vi "Initialize Connection.vi"(8 "error in (no error)":errorcluster, 9 "GUID":string, 10 "TCP Timeout":i32, 11 "TCP Connection":refnum<k5>) -> (0 "error out":errorcluster, 3 "tWorkerTCPConnection out":refnum<class "tWorkerTCPConnection.lvclass">)   [LabVIEW 2013, in "tWorkerTCPConnection.lvlib" / "tWorkerTCPConnection.lvclass"]
uses:
  tWorkerTCPConnection.lvclass
  tWorkerTCPConnection.lvclass/tWorkerTCPConnection.ctl
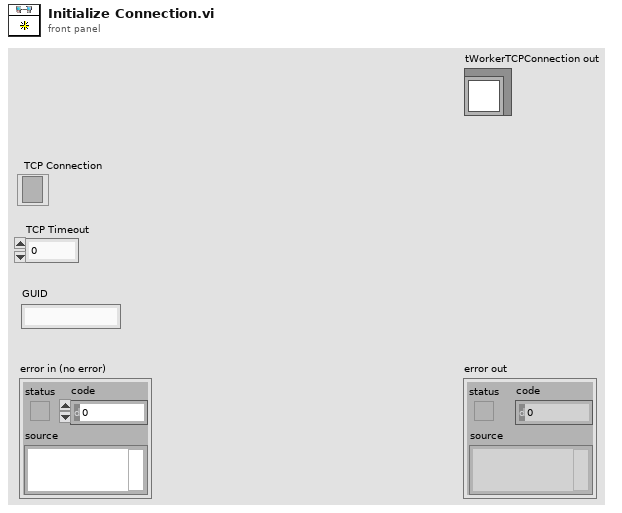
[diagram p1: front panel]
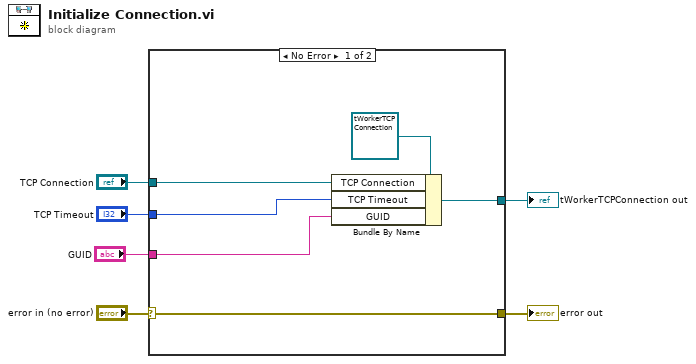
[diagram p0: block diagram]
diagram:
  n1 = case shown="No Error" "error in (no error)" {
    selector: "error in (no error)" -> [w10 w13]
    tunnel: [w10 w13] -> w5
    tunnel: "TCP Connection" -> [w9 _]
    tunnel: [w11 _] -> w3
    tunnel: "TCP Timeout" -> [w8 _]
    tunnel: "GUID" -> [w7 _]
    frame No Error {
      n2 = Bundle By Name(cluster=refnum<class "tWorkerTCPConnection.lvclass"> refnum ("tWorkerTCPConnection out"), "TCP Connection"=w9, "TCP Timeout"=w8, "GUID"=w7) -> (w11:refnum<class "tWorkerTCPConnection.lvclass">)
    }
    frame Error {
    }
  }
  "error out" <- w5
  "tWorkerTCPConnection out" <- w3
